vi "CreateWfrm.vi"(8 "ErrorArray In":errorcluster[](array[cluster]), 10 "clFrontPanelControlRefs":T1, 11 "NISTBus In":refnum<class "NISTBus.lvclass">) -> (0 "ErrorArray Out":errorcluster[](array[cluster]), 3 "NISTBus Out":refnum<class "NISTBus.lvclass">)   [LabVIEW 2014, in "Bus.lvlib" / "NISTBus.lvclass"]
uses:
  NISTBus.lvclass
  WfrmGenerator/WfrmModule/WfrmModule.lvlib
  <userlib>/NIST/NISTErrorLib/NISTErrorLib.lvlib
  FGenPlugins/MyPluginBaseClass/TypeDef/PluginParams.ctl
  FGenPlugins/MyPluginBaseClass/NISTFGenPluginsBase.lvclass
  WfrmGenerator/WfrmPlugins/EventPluginBaseClass/TypeDefs/dblEvtSignalArray.ctl
  WfrmGenerator/WfrmPlugins/EventPluginBaseClass/BaseWfrmPlugin.lvclass
  FGenPlugins/MyPluginBaseClass/TypeDef/CreateArbWfrmParams.ctl
  WfrmGenerator/WfrmPlugins/EventPluginBaseClass/TypeDefs/clEvtConfig.ctl
  WfrmGenerator/WfrmModule/PublicAPI/Arguments/Requests/dblEvtParams.ctl
  Framework/FrontPanel/TypeDefs/clFrontPanelControlRefs.ctl
  Framework/TestFramework.lvlib
  FGenPlugins/MyPluginBaseClass/TypeDef/ConfigArbWfrmParams.ctl
  FGenPlugins/MyPluginBaseClass/TypeDef/TriggerParams.ctl
panel:
  # "When you add a control \non the front panel, add a\nreference for it in this\ntype def.  This cluster\nwill hold all of the refer-\nences to the front panel\ncontrols in order to pass\nthese control references \nto subvis."
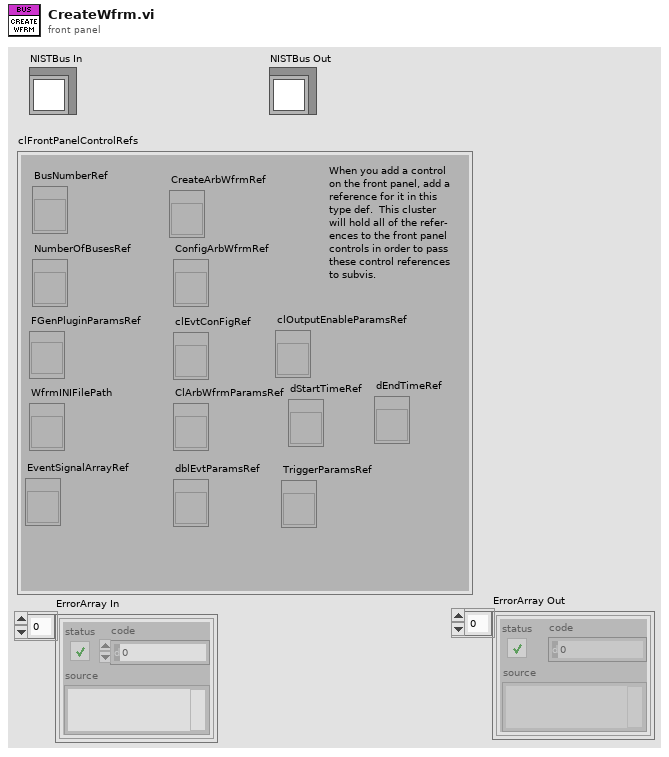
[diagram p1: front panel]
types:
  T1 = typedef "TestFramework.lvlib/clFrontPanelControlRefs.ctl" = cluster{"BusNumberRef":refnum<vi>, "NumberOfBusesRef":refnum<vi>, "FGenPluginParamsRef":refnum<vi>, "WfrmINIFilePath":refnum<vi>, "EventSignalArrayRef":refnum<vi>, "CreateArbWfrmRef":refnum<vi>, "clEvtConFigRef":refnum<vi>, "dblEvtParamsRef":refnum<vi>, "clOutputEnableParamsRef":refnum<vi>, "ConfigArbWfrmRef":refnum<vi>, "ClArbWfrmParamsRef":refnum<vi>, "dStartTimeRef":refnum<vi>, "dEndTimeRef":refnum<vi>, "TriggerParamsRef":refnum<vi>}
  T2 = typedef "NISTWfrmPlugins.lvlib/EventPluginBaseClass.lvclass/clEvtConfig.ctl" = cluster{"T0(UTC)":dbl, "F0":dbl, "Fs":i32, "FSamp":u32}
  T3 = typedef "NISTWfrmModule.lvlib/dblEvtParams.ctl" = dbl[][]
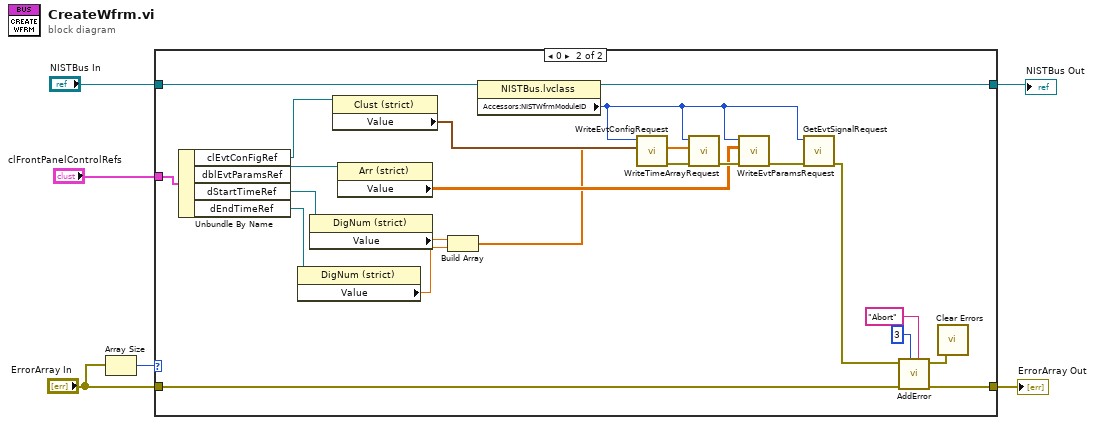
[diagram p0: block diagram]
diagram:
  n1 = Array Size(array="ErrorArray In") -> (size(s)=w6:i32)
  n2 = case shown="0" w6 {
    tunnel: "ErrorArray In" -> [w8 w23]
    tunnel: "NISTBus In" -> [w7 w30]
    tunnel: [w8 w24] -> w3
    tunnel: [w7 w22] -> w2
    tunnel: "clFrontPanelControlRefs" -> [_ w18]
    frame 1, Default {
    }
    frame 0 {
      n3 = Unbundle By Name(w18) -> ("clEvtConFigRef"=w17:refnum<vi>, "dblEvtParamsRef"=w15:refnum<vi>, "dStartTimeRef"=w13:refnum<vi>, "dEndTimeRef"=w11:refnum<vi>)
      n4 = property class="DigNum (strict)"(reference=w11) -> ("Value"=w10:dbl)  [unwired: 1 in, 2 out]
      n5 = property class="DigNum (strict)"(reference=w13) -> ("Value"=w12:dbl)  [unwired: 1 in, 2 out]
      n6 = property class="Clust (strict)"(reference=w17) -> ("Value"=w16:T2)  [unwired: 1 in, 2 out]
      n7 = property class="Arr (strict)"(reference=w15) -> ("Value"=w14:T3)  [unwired: 1 in, 2 out]
      n8 = Build Array(w12, w10) -> (w9:dbl[])
      n9 = property class="NISTBus.lvclass"(reference=w30) -> (reference out=w22:refnum<class "NISTBus.lvclass">, "Accessors:NISTWfrmModuleID"=w20:i32)  [unwired: 1 in, 1 out]
      n10 = call "WriteEvtConfigRequest.vi"("clEvtConfig"=w16, "ModuleID"=w20) -> ("error out"=w29:errorcluster)  [unwired: 9 in]
      n11 = call "WriteTimeArrayRequest.vi"("error in (no error)"=w29, "clTimeParams"=w9, "ModuleID"=w20) -> ("error out"=w28:errorcluster)  [unwired: 8 in]
      n12 = call "WriteEvtParamsRequest.vi"("error in (no error)"=w28, "EvtParams"=w14, "ModuleID"=w20) -> ("error out"=w21:errorcluster)  [unwired: 8 in]
      n13 = call "GetEvtSignalRequest.vi"("error in (no error)"=w21, "ModuleID"=w20) -> ("error out"=w19:errorcluster)  [unwired: 9 in]
      n14 = call <userlib>:"AddError.vi"("Severity"="Abort" ("String"), "Priority"=u8 3, "ErrorArray"=w23, "error in (no error)"=w19) -> ("ErrorArray"=w24:errorcluster[], "error out"=w25:errorcluster)  [unwired: 6 in]
      n15 = call <vilib>:"Clear Errors.vi"("error in (no error)"=w25) -> ()  [unwired: 5 in, 2 out]
    }
  }
  "ErrorArray Out" <- w3
  "NISTBus Out" <- w2
